vi "symulacja_mikroskopu_Karol_Wrzesiński.vi"() -> ()   [LabVIEW 2020]
uses:
  <vilib>/Utility/file.llb/Write Delimited Spreadsheet (DBL).vi
panel:
  in  "wiązki biegnące w mikroskopie\nskala 1pixel=1mm^2":picture
  in  "Add Button":bool
  out "error out":errorcluster
  in  "?":bool
  in  "zapisz wykres":bool
  out "XY Graph":cluster{dbl, dbl}[](graph)
  in  "zapisz pomiary":bool
  out "?":dbl[](array[numeric])
  out "rozdzielczosc optyczna":dbl
  out "apertura":dbl
  out "powieksznie calkowite":dbl
  out "powieksznie obiektywu":dbl
  out "powieksznie okularu":dbl
  in  "ogniskowa okularu[mm]":dbl
  in  "ogniskowa obiektywu[mm]":dbl
  in  "L-odleglosc miedzy\nogniskowymi soczewek[mm]":dbl
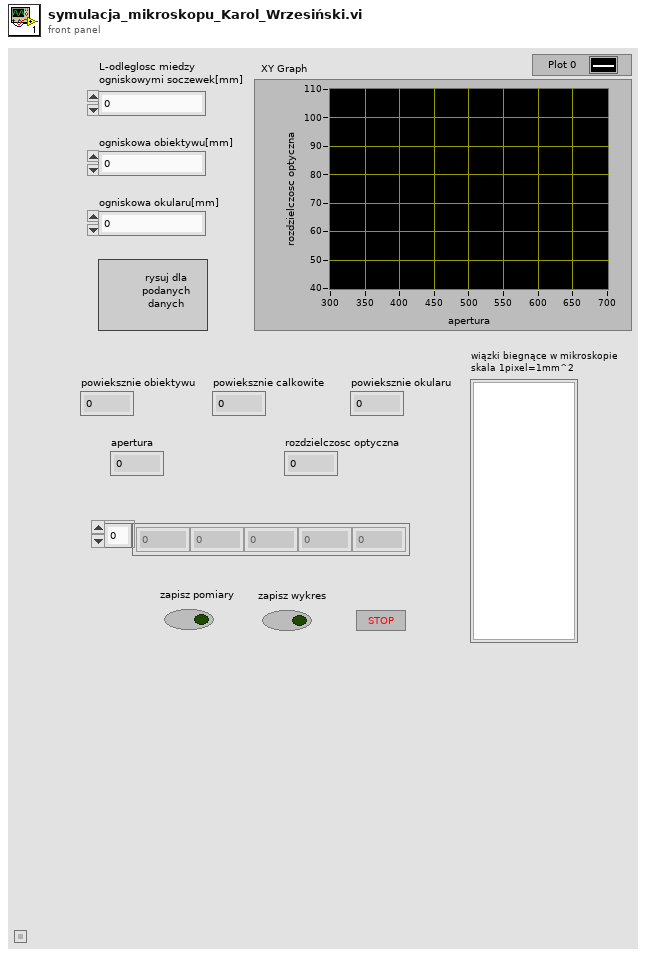
[diagram p1: front panel]
types:
  T1 = cluster{"Width":u16, "Style":enum32{"Solid", "Dash", "Dot", "DashDot", "DashDotDot"}}
  T2 = typedef "imagedata.ctl" = cluster{"image type":i32, "image depth":i32, "image":u8[], "mask":u8[], "colors":u32[], "Rectangle":cluster{"left":i16, "top":i16, "right":i16, "bottom":i16}}
  T3 = cluster{"powieksznie obiektywu":dbl, "powieksznie okularu ":dbl, "powieksznie calkowite":dbl, "apertura":dbl, "rozdzielczosc optyczna":dbl}
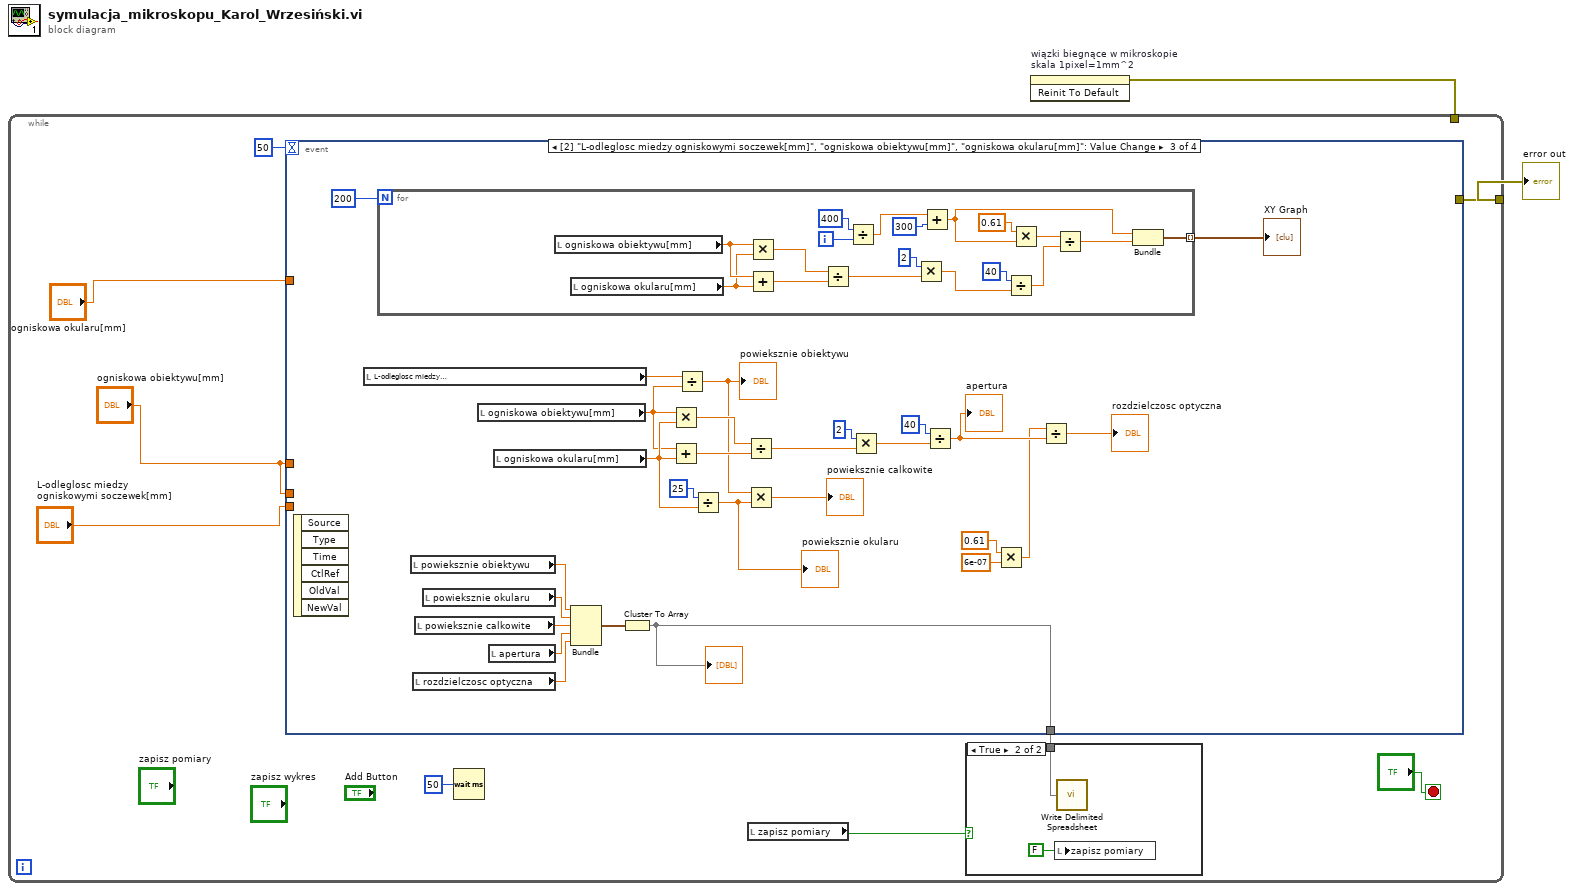
[diagram p0: block diagram]
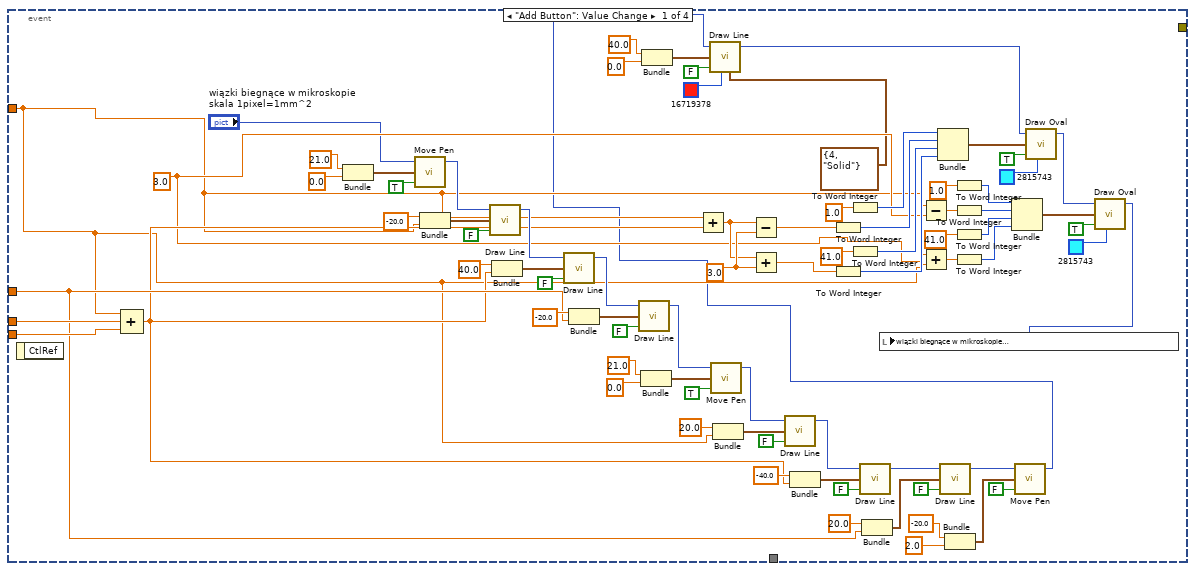
[diagram p3: hidden frame]
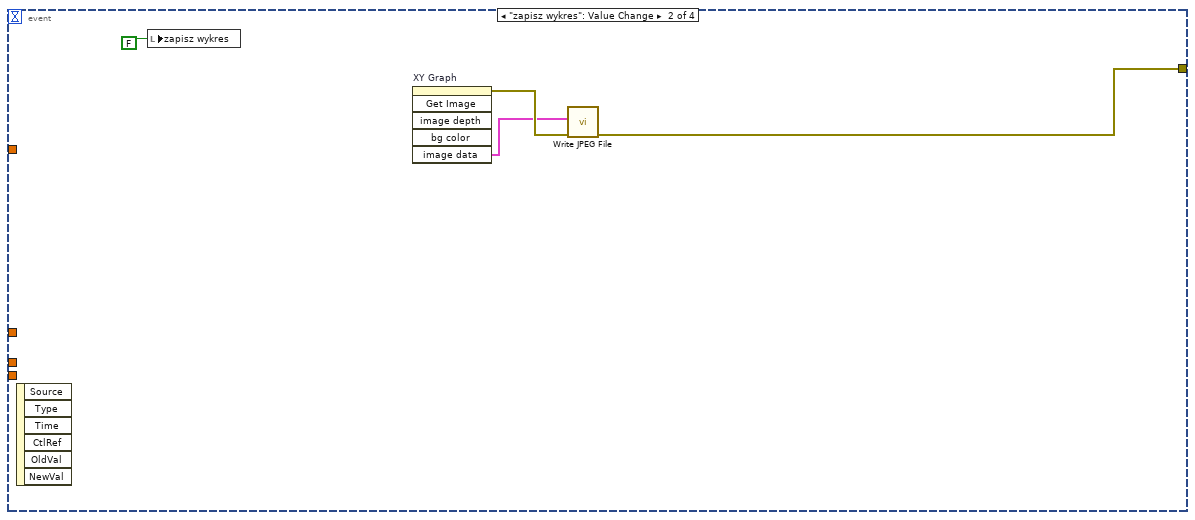
[diagram p4: hidden frame]
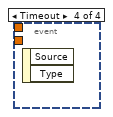
[diagram p5: hidden frame]
diagram:
  n1 = invoke on="wiązki biegnące w mikroskopie\nskala 1pixel=1mm^2" class="Pict" method="Reinit To Default"() -> (error out=w1:errorcluster)  [unwired: 3 in, 2 out]
  n2 = while {
    tunnel: [w8] -> w2
    tunnel: w1 -> [_]
    stop <- "?" stop-if-true
    n3 = event shown="[2] \"L-odleglosc miedzy ogniskowymi soczewek[mm]\", \"ogniskowa obiektywu[mm]\", \"ogniskowa okularu[mm]\": Value Change" {
      selector: _ -> [_ _ _ _]
      dyn-events: _ -> [_ _ _ _]
      timeout: 50 -> [_ _ _ _]
      tunnel: "ogniskowa okularu[mm]" -> [w29 _ _ _]
      tunnel: "ogniskowa obiektywu[mm]" -> [w82 _ _ _]
      tunnel: "L-odleglosc miedzy\nogniskowymi soczewek[mm]" -> [w81 _ _ _]
      tunnel: "ogniskowa obiektywu[mm]" -> [w63 _ _ _]
      tunnel: [_ w94 _ _] -> w8
      tunnel: [_ _ w97 _] -> w3
      event "Add Button": Value Change {
        w38 = 3.0
        w52 = 3.0
        n4 = event-data() -> ()  [unwired: 1 in, 1 out]
        n5 = Compound Arithmetic op=ADD(w29, w82, w81) -> (w44:dbl)
        n6 = Bundle(21.0, 0.0) -> (w92:cluster{dbl, dbl})  [unwired: 1 in]
        n7 = call <vilib>:"Move Pen.vi"("absolute coordinates?(T)"=TRUE, "new position"=w92, "picture"="wiązki biegnące w mikroskopie\nskala 1pixel=1mm^2") -> ("new picture"=w88:picture)  [unwired: 2 in]
        n8 = Bundle(-20.0, "ogniskowa okularu[mm]"=w29) -> (w86:cluster{dbl, "ogniskowa okularu[mm]":dbl})  [unwired: 1 in]
        n9 = call <vilib>:"Draw Line.vi"("picture"=w88, "end point"=w86, "absolute coordinates?(T)"=FALSE) -> ("new picture"=w83:picture)  [unwired: 6 in]
        n10 = Bundle(40.0, w44) -> (w84:cluster{dbl, dbl})  [unwired: 1 in]
        n11 = call <vilib>:"Draw Line.vi"("picture"=w83, "end point"=w84, "absolute coordinates?(T)"=FALSE) -> ("new picture"=w80:picture)  [unwired: 6 in]
        n12 = Bundle(-20.0, "ogniskowa obiektywu[mm]"=w63) -> (w78:cluster{dbl, "ogniskowa obiektywu[mm]":dbl})  [unwired: 1 in]
        n13 = call <vilib>:"Draw Line.vi"("picture"=w80, "end point"=w78, "absolute coordinates?(T)"=FALSE) -> ("new picture"=w60:picture)  [unwired: 6 in]
        n14 = Bundle(21.0, 0.0) -> (w59:cluster{dbl, dbl})  [unwired: 1 in]
        n15 = Bundle(40.0, 0.0) -> (w20:cluster{dbl, dbl})  [unwired: 1 in]
        n16 = Add(x=w29, y=w44) -> (x+y=w43:dbl)
        n17 = call <vilib>:"Move Pen.vi"("absolute coordinates?(T)"=TRUE, "new position"=w59, "picture"=w60) -> ("new picture"=w57:picture)  [unwired: 2 in]
        n18 = Bundle(20.0, "ogniskowa okularu[mm]"=w29) -> (w72:cluster{dbl, "ogniskowa okularu[mm]":dbl})  [unwired: 1 in]
        n19 = Subtract(x=w43, y=w52) -> (x-y=w49:dbl)
        n20 = Add(x=w43, y=w52) -> (x+y=w47:dbl)
        n21 = call <vilib>:"Draw Line.vi"("picture"=w57, "end point"=w72, "absolute coordinates?(T)"=FALSE) -> ("new picture"=w68:picture)  [unwired: 6 in]
        n22 = Bundle(-40.0, w44) -> (w70:cluster{dbl, dbl})  [unwired: 1 in]
        n23 = To Word Integer(number=w49) -> (16bit integer=w48:i16)
        n24 = To Word Integer(number=w47) -> (16bit integer=w46:i16)
        n25 = To Word Integer(number=1.0) -> (16bit integer=w54:i16)
        n26 = To Word Integer(number=41.0) -> (16bit integer=w45:i16)
        n27 = call <vilib>:"Draw Line.vi"("picture"=w68, "end point"=w70, "absolute coordinates?(T)"=FALSE) -> ("new picture"=w65:picture)  [unwired: 6 in]
        n28 = Bundle(20.0, "ogniskowa obiektywu[mm]"=w63) -> (w66:cluster{dbl, "ogniskowa obiektywu[mm]":dbl})  [unwired: 1 in]
        n29 = Subtract(x=w29, y=w38) -> (x-y=w35:dbl)
        n30 = Add(x=w29, y=w38) -> (x+y=w33:dbl)
        n31 = Bundle(w54, w48, w45, w46) -> (w56:cluster{i16, i16, i16, i16})  [unwired: 1 in]
        n32 = call <vilib>:"Draw Line.vi"("picture"=w65, "end point"=w66, "absolute coordinates?(T)"=FALSE) -> ("new picture"=w28:picture)  [unwired: 6 in]
        n33 = Bundle(-20.0, 2.0) -> (w26:cluster{dbl, dbl})  [unwired: 1 in]
        n34 = To Word Integer(number=1.0) -> (16bit integer=w40:i16)
        n35 = To Word Integer(number=w35) -> (16bit integer=w34:i16)
        n36 = To Word Integer(number=41.0) -> (16bit integer=w31:i16)
        n37 = To Word Integer(number=w33) -> (16bit integer=w32:i16)
        n38 = Bundle(w40, w34, w31, w32) -> (w42:cluster{i16, i16, i16, i16})  [unwired: 1 in]
        n39 = call <vilib>:"Move Pen.vi"("absolute coordinates?(T)"=FALSE, "new position"=w26, "picture"=w28) -> ("new picture"=w15:picture)  [unwired: 2 in]
        n40 = call <vilib>:"Draw Line.vi"("picture"=w15, "end point"=w20, "absolute coordinates?(T)"=FALSE, "color(black)"=u32 16719378, "pen"=T1 {"Width"=4, "Style"=enum."Solid"}) -> ("new picture"=w23:picture)  [unwired: 4 in]
        n41 = call <vilib>:"Draw Oval.vi"("picture"=w23, "rect"=w56, "fill?(F)"=TRUE, "color(black)"=u32 2815743) -> ("new picture"=w30:picture)  [unwired: 5 in]
        n42 = call <vilib>:"Draw Oval.vi"("picture"=w30, "rect"=w42, "fill?(F)"=TRUE, "color(black)"=u32 2815743) -> ("new picture"=w14:picture)  [unwired: 5 in]
        n43 = local write "wiązki biegnące w mikroskopie\nskala 1pixel=1mm^2"(w14) -> ()
      }
      event "zapisz wykres": Value Change {
        n44 = event-data() -> ()  [unwired: 1 in, 6 out]
        n45 = local write "zapisz wykres"(FALSE) -> ()
        n46 = invoke on="XY Graph" class="XYGraph (strict)" method="Get Image"() -> (error out=w96:errorcluster, "image data"=w95:T2)  [unwired: 6 in, 4 out]
        n47 = call <vilib>:"Write JPEG File.vi"("error in (no error)"=w96, "image data"=w95) -> ("error out"=w94:errorcluster)  [unwired: 8 in, 1 out]
      }
      event "L-odleglosc miedzy\nogniskowymi soczewek[mm]", "ogniskowa obiektywu[mm]", "ogniskowa okularu[mm]": Value Change {
        n48 = event-data() -> ()  [unwired: 1 in, 6 out]
        n49 = local read "L-odleglosc miedzy\nogniskowymi soczewek[mm]"() -> (w109:dbl)
        n50 = for {
          N: 200 -> [_]
          tunnel: [w138] -> w123 mode=indexing
          i -> [w136]
          n51 = local read "ogniskowa obiektywu[mm]"() -> (w128:dbl)
          n52 = local read "ogniskowa okularu[mm]"() -> (w127:dbl)
          n53 = Multiply(x=w128, y=w127) -> (x*y=w131:dbl)
          n54 = Add(x=w128, y=w127) -> (x+y=w132:dbl)
          n55 = Divide(x=w131, y=w132) -> (x/y=w130:dbl)
          n56 = Divide(x=400, y=w136) -> (x/y=w126:dbl)
          n57 = Multiply(x=2, y=w130) -> (x*y=w134:dbl)
          n58 = Add(x=w126, y=300) -> (x+y=w124:dbl)
          n59 = Divide(x=40, y=w134) -> (x/y=w129:dbl)
          n60 = Multiply(x=0.61, y=w124) -> (x*y=w139:dbl)
          n61 = Divide(x=w139, y=w129) -> (x/y=w137:dbl)
          n62 = Bundle(w124, w137) -> (w138:cluster{dbl, dbl})  [unwired: 1 in]
        }
        "XY Graph" <- w123
        n63 = local read "powieksznie obiektywu"() -> (w102:dbl)
        n64 = local read "rozdzielczosc optyczna"() -> (w98:dbl)
        n65 = local read "powieksznie calkowite"() -> (w100:dbl)
        n66 = local read "powieksznie okularu"() -> (w101:dbl)
        n67 = local read "ogniskowa obiektywu[mm]"() -> (w119:dbl)
        n68 = local read "apertura"() -> (w99:dbl)
        n69 = local read "ogniskowa okularu[mm]"() -> (w120:dbl)
        n70 = Bundle("powieksznie obiektywu"=w102, "powieksznie okularu"=w101, "powieksznie calkowite"=w100, "apertura"=w99, "rozdzielczosc optyczna"=w98) -> (w103:T3)  [unwired: 1 in]
        n71 = Cluster To Array(cluster=w103) -> (array=w97:dbl[])
        "?" <- w97
        n72 = Multiply(x=w119, y=w120) -> (x*y=w117:dbl)
        n73 = Add(x=w119, y=w120) -> (x+y=w116:dbl)
        n74 = Divide(x=w109, y=w119) -> (x/y=w112:dbl)
        "powieksznie obiektywu" <- w112
        n75 = Divide(x=25, y=w120) -> (x/y=w111:dbl)
        "powieksznie okularu" <- w111
        n76 = Divide(x=w117, y=w116) -> (x/y=w118:dbl)
        n77 = Multiply(x=w112, y=w111) -> (x*y=→"powieksznie calkowite":dbl)
        n78 = Multiply(x=2, y=w118) -> (x*y=w115:dbl)
        n79 = Divide(x=40, y=w115) -> (x/y=w121:dbl)
        "apertura" <- w121
        n80 = Multiply(x=0.61, y=6e-07) -> (x*y=w113:dbl)
        n81 = Divide(x=w113, y=w121) -> (x/y=→"rozdzielczosc optyczna":dbl)
      }
      event Timeout {
        n82 = event-data() -> ()  [unwired: 1 in, 2 out]
      }
    }
    n83 = Wait (ms)(milliseconds to wait=u32 50) -> ()  [unwired: 1 out]
    n84 = local read "zapisz pomiary"() -> (w4:bool)
    n85 = case shown="True" w4 {
      tunnel: w3 -> [_ w12]
      frame False {
      }
      frame True {
        n86 = local write "zapisz pomiary"(FALSE) -> ()
        n87 = call-poly <vilib>:"Write Delimited Spreadsheet.vi"("1D data"=w12) -> ()  [unwired: 13 in, 2 out]
      }
    }
  }
  "error out" <- w2
